vi "Tone RMS from Mag Spec (2D).vi"(9 "Frequency (kHz)":dbl[](array[numeric]), 10 "df (kHz)":dbl, 11 "Magnitude (dB)":dbl[](array[numeric])) -> (1 "Fpeak (kHz)":dbl[](array[numeric]), 2 "RMS (dB)":dbl[](array[numeric]), 3 "RMS (V)":dbl[](array[numeric]))   [LabVIEW 2020]
uses:
  Linear to dB (array).vi
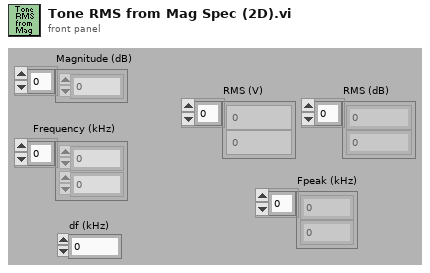
[diagram p1: front panel]
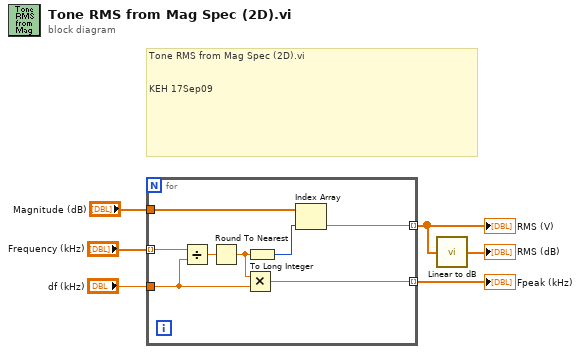
[diagram p0: block diagram]
diagram:
  # "Tone RMS from Mag Spec (2D).vi\n\n\nKEH 17Sep09"
  n1 = for {
    tunnel: "df (kHz)" -> [w9]
    tunnel: "Frequency (kHz)" -> [w14] mode=indexing
    tunnel: "Magnitude (dB)" -> [w12]
    tunnel: [w7] -> w4 mode=indexing
    tunnel: [w8] -> w2 mode=indexing
    n2 = Divide(x=w14, y=w9) -> (x/y=w13:dbl)
    n3 = Round To Nearest(number=w13) -> (nearest integer value=w10:dbl)
    n4 = Multiply(x=w10, y=w9) -> (x*y=w8:dbl)
    n5 = To Long Integer(number=w10) -> (32bit integer=w11:i32)
    n6 = Index Array(array=w12, index=w11) -> (element=w7:dbl)
  }
  "RMS (V)" <- w4
  "Fpeak (kHz)" <- w2
  n7 = call-poly "Linear to dB.vi"("linear"=w4) -> ("dB"=→"RMS (dB)":dbl[])
